vi "Proyecto Final.vi"() -> ()   [LabVIEW 2014]
panel:
  out "2061":string
  out "2060":string
  out "2059":string
  out "Datos Ambos":string
  out "Datos 2":string
  out "Datos 1":string
  in  "Modo":i16(slide) scale=1.0..5.0
  out "Motor 5":i64
  out "Motor 6":i64
  out "Motor 4":i64
  out "Motor 3":i64
  out "Motor 2":i64
  out "Motor 1":i64
  in  "reset":bool
  in  "?":bool
  in  "Motor 6":i64(knob) scale=-500.0..500.0
  in  "Motor 5":i64(knob) scale=-500.0..500.0
  in  "Motor 4":i64(knob) scale=-500.0..500.0
  in  "Motor 3":i64(knob) scale=-500.0..500.0
  in  "Motor 2":i64(knob) scale=-500.0..500.0
  in  "Motor 1":i64(knob) scale=-500.0..500.0
  # "Instrucciones:\nEn esta pantalla se pueden observar\n6 perillas, 6 indicadores y una barra \npara seleccionar el modo.\n\nBarra de Seleccion de Modo\nBrazo A LM: El leap motion enviara \nvalores del 0 al 5 para escoger una\nrutina predefinida en el brazo A\n\nBrazo B LM: El leap motion enviara \nvalores del 0 al 5 para escoger una\nrutina predefinida en el brazo B\n\nAmbos: Se controlaran ambos brazos\nal mismo tiempo\n\nBrazo A Manual: El brazo A tomará la\nposición que tengan las perillas\n\nBrazo B Manual: El brazo B tomará la\nposición que tengan las perillas"
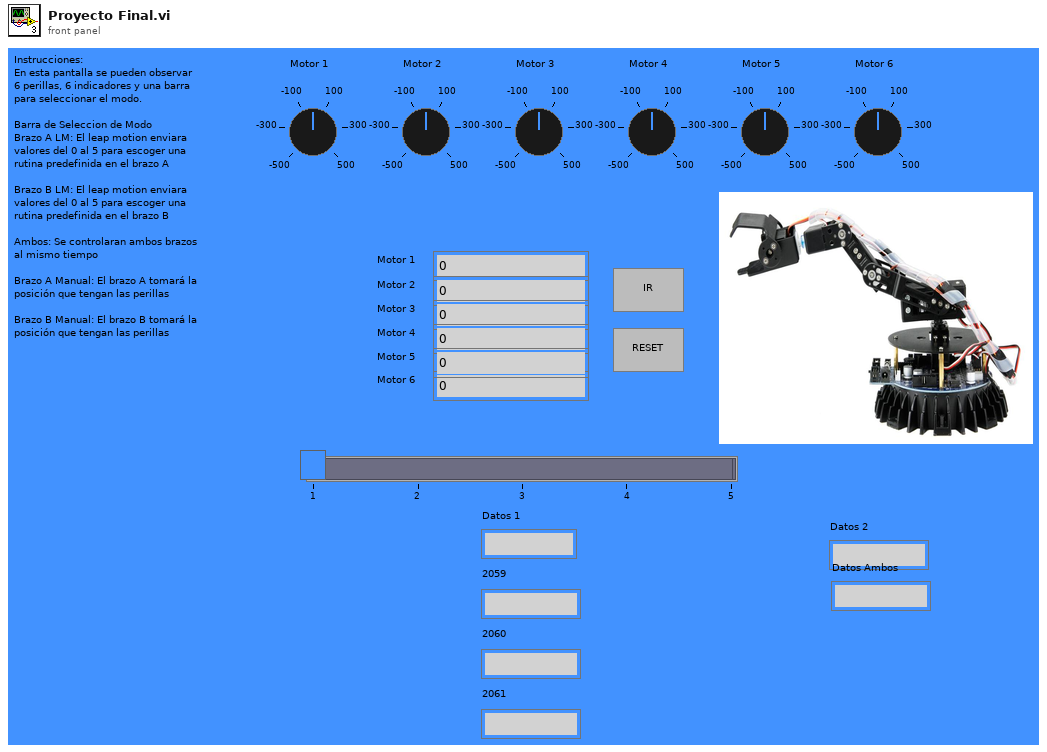
[diagram p1: front panel]
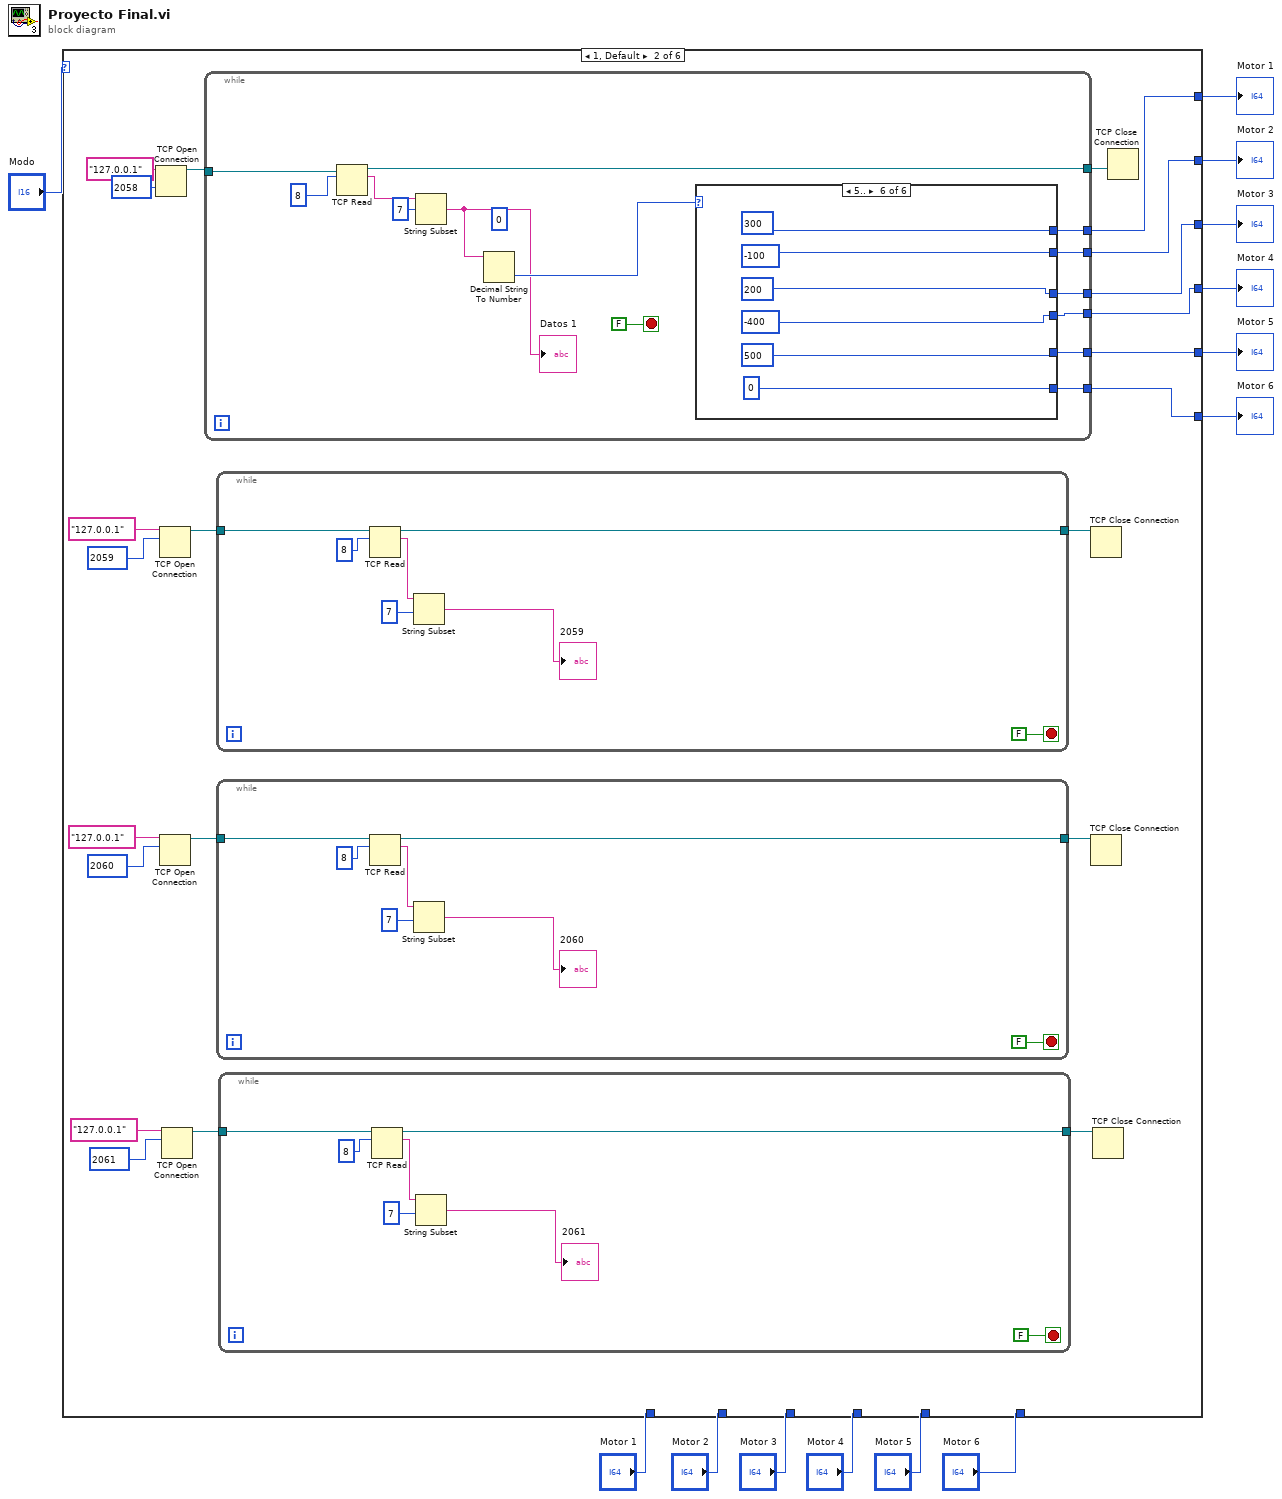
[diagram p0: block diagram]
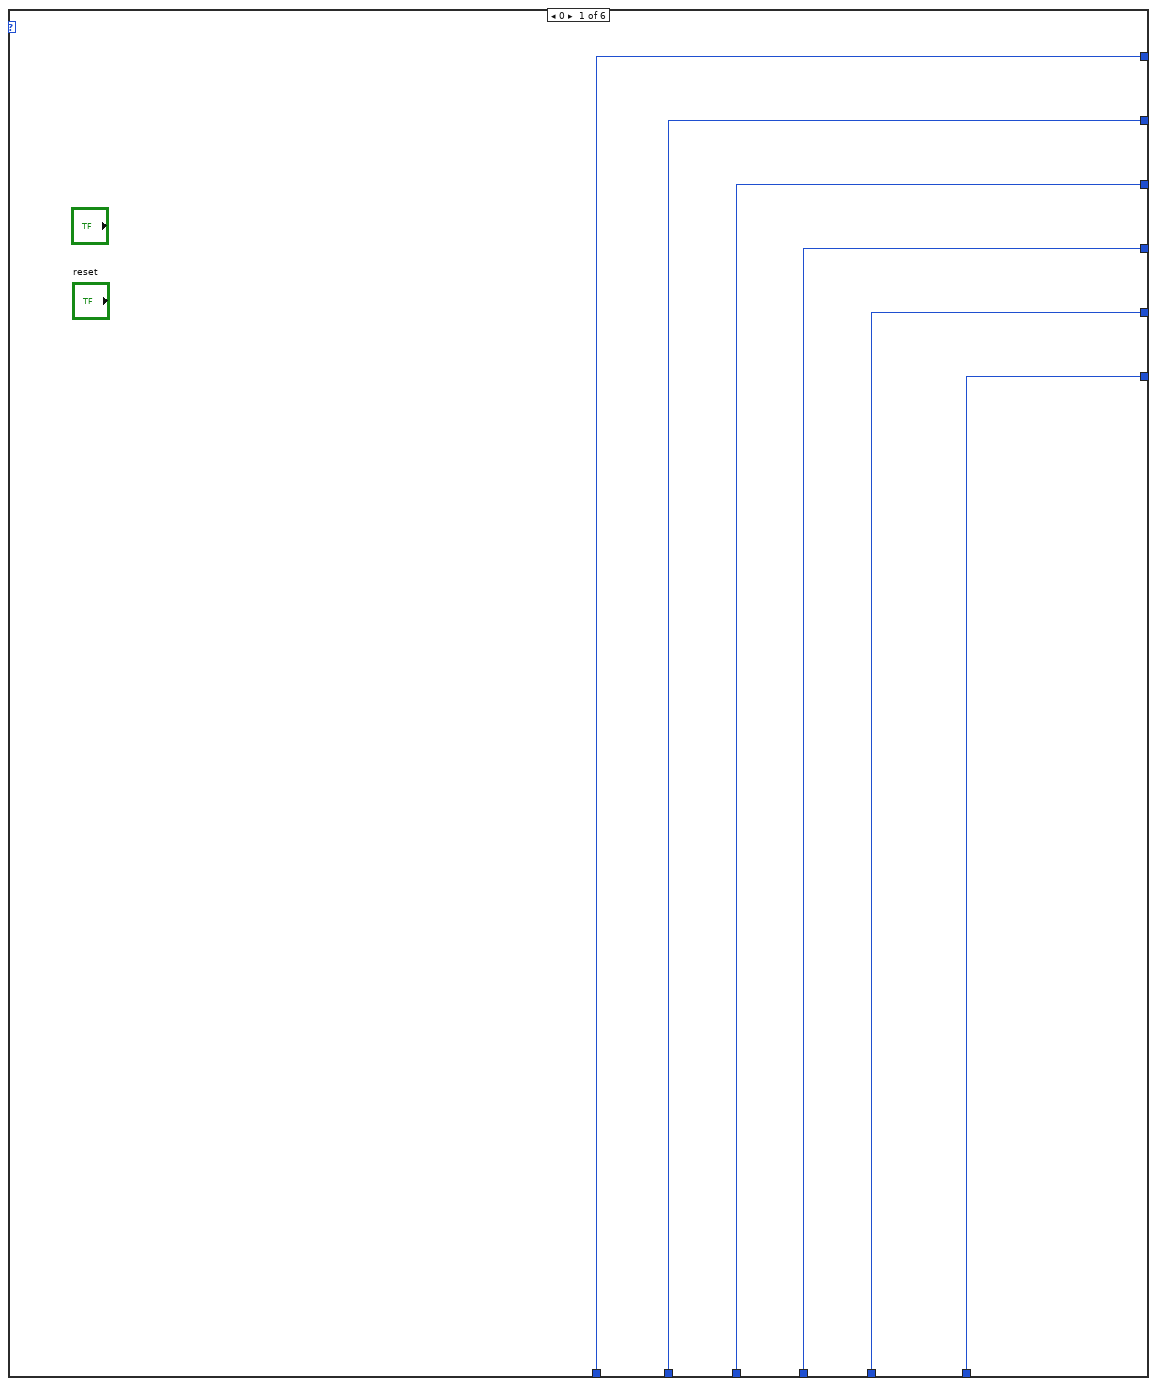
[diagram p2: hidden frame]
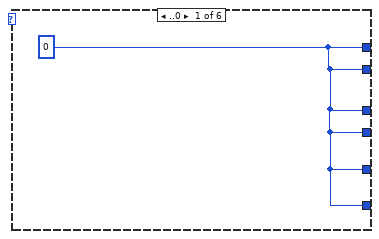
[diagram p3: hidden frame]
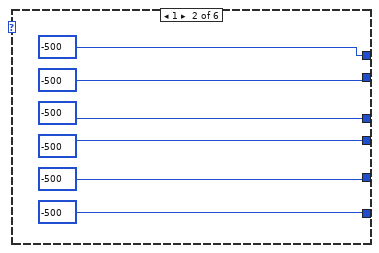
[diagram p4: hidden frame]
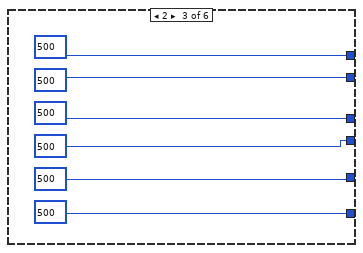
[diagram p5: hidden frame]
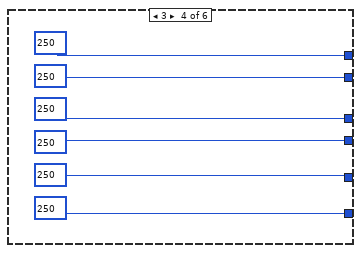
[diagram p6: hidden frame]
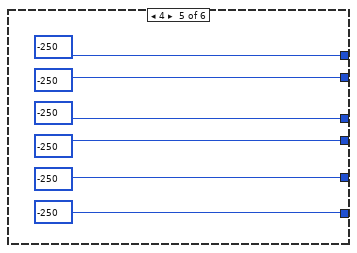
[diagram p7: hidden frame]
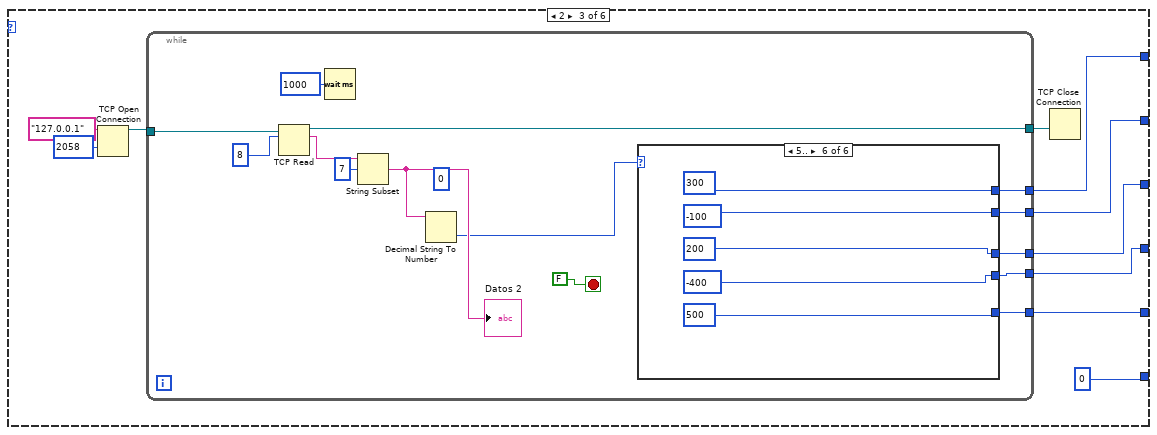
[diagram p8: hidden frame]
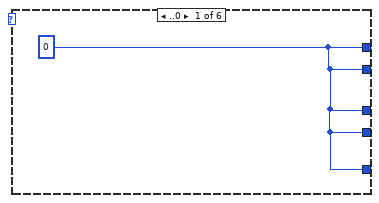
[diagram p9: hidden frame]
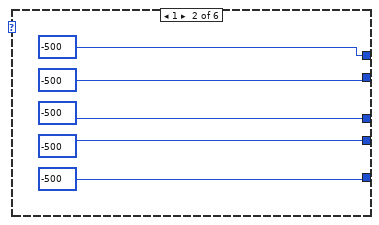
[diagram p10: hidden frame]
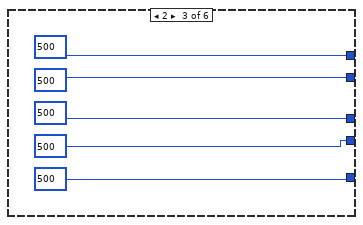
[diagram p11: hidden frame]
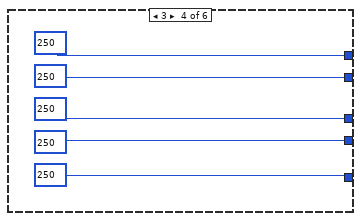
[diagram p12: hidden frame]
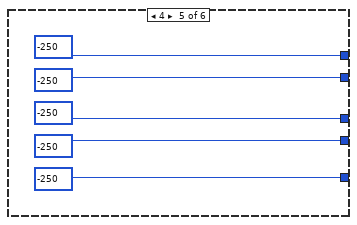
[diagram p13: hidden frame]
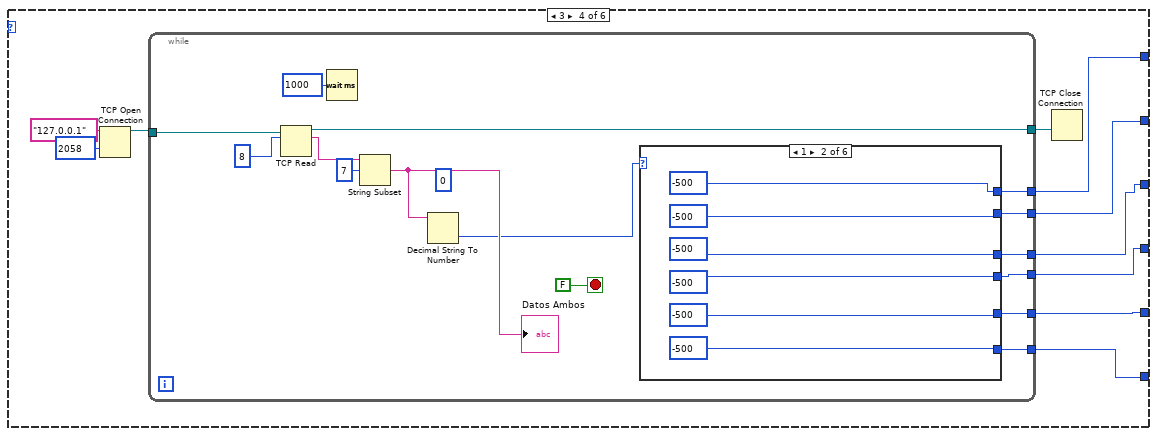
[diagram p14: hidden frame]
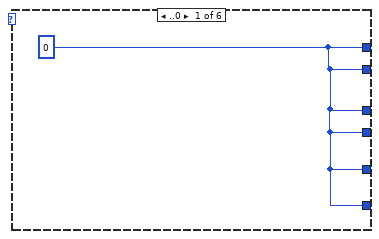
[diagram p15: hidden frame]
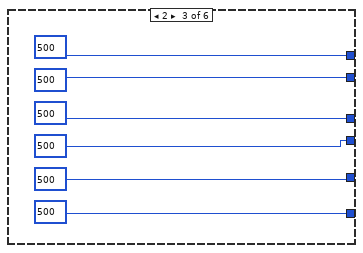
[diagram p16: hidden frame]
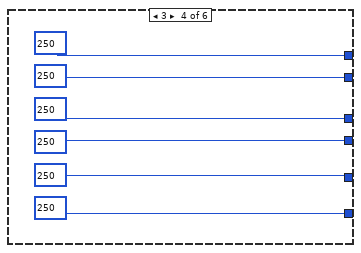
[diagram p17: hidden frame]
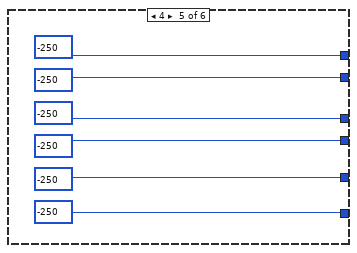
[diagram p18: hidden frame]
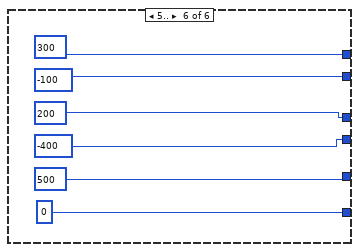
[diagram p19: hidden frame]
diagram:
  n1 = case shown="1, Default" "Modo" {
    tunnel: [w19 w37 w113 w163 w219 w225] -> w13
    tunnel: [w18 w36 w112 w162 w218 w224] -> w12
    tunnel: [w17 w35 w111 w161 w217 w223] -> w11
    tunnel: [w16 w34 w110 w160 w216 w222] -> w10
    tunnel: [w15 w33 w109 w159 w215 w221] -> w9
    tunnel: [w14 w32 0 w158 w214 0] -> w8
    tunnel: "Motor 1" -> [w19 _ _ _ w219 w225]
    tunnel: "Motor 2" -> [w18 _ _ _ w218 w224]
    tunnel: "Motor 3" -> [w17 _ _ _ w217 w223]
    tunnel: "Motor 4" -> [w16 _ _ _ w216 w222]
    tunnel: "Motor 5" -> [w15 _ _ _ w215 w221]
    tunnel: "Motor 6" -> [w14 _ _ _ w214 _]
    frame 0 {
    }
    frame 1, Default {
      n2 = TCP Open Connection(address="127.0.0.1", remote port or service name=u16 2058) -> (connection ID=w41:refnum<k5>)  [unwired: 3 in, 1 out]
      n3 = TCP Open Connection(address="127.0.0.1", remote port or service name=u16 2059) -> (connection ID=w29:refnum<k5>)  [unwired: 3 in, 1 out]
      n4 = TCP Open Connection(address="127.0.0.1", remote port or service name=u16 2060) -> (connection ID=w26:refnum<k5>)  [unwired: 3 in, 1 out]
      n5 = TCP Open Connection(address="127.0.0.1", remote port or service name=u16 2061) -> (connection ID=w21:refnum<k5>)  [unwired: 3 in, 1 out]
      n6 = while {
        tunnel: w41 -> [w76]
        tunnel: [w74] -> w38
        tunnel: [w71] -> w37
        tunnel: [w70] -> w36
        tunnel: [w69] -> w35
        tunnel: [w68] -> w34
        tunnel: [w67] -> w33
        tunnel: [w66] -> w32
        stop <- FALSE stop-if-true
        (unwired) 0 ("offset (0)")
        n7 = TCP Read(connection ID=w76, bytes to read=8) -> (connection ID out=w74:refnum<k5>, data out=w72:string)  [unwired: 3 in, 1 out]
        n8 = String Subset(string=w72, offset (0)=7) -> (substring=w64:string)  [unwired: 1 in]
        "Datos 1" <- w64
        n9 = Decimal String To Number(string=w64) -> (number=w65:i32)  [unwired: 2 in, 1 out]
        n10 = case shown="5.." w65 {
          tunnel: [w77 -500 500 250 -250 300] -> w71
          tunnel: [w77 -500 500 250 -250 -100] -> w70
          tunnel: [w77 -500 500 250 -250 200] -> w69
          tunnel: [w77 -500 500 250 -250 -400] -> w68
          tunnel: [w77 -500 500 250 -250 500] -> w67
          tunnel: [w77 -500 500 250 -250 0] -> w66
          frame ..0 {
            w77 = 0
          }
          frame 1 {
          }
          frame 2 {
          }
          frame 3 {
          }
          frame 4 {
          }
          frame 5.. {
          }
        }
      }
      n11 = while {
        tunnel: w29 -> [w62]
        tunnel: [w61] -> w28
        stop <- FALSE stop-if-true
        n12 = TCP Read(connection ID=w62, bytes to read=8) -> (connection ID out=w61:refnum<k5>, data out=w57:string)  [unwired: 3 in, 1 out]
        n13 = String Subset(string=w57, offset (0)=7) -> (substring=→"2059":string)  [unwired: 1 in]
      }
      n14 = while {
        tunnel: w26 -> [w55]
        tunnel: [w54] -> w27
        stop <- FALSE stop-if-true
        n15 = TCP Read(connection ID=w55, bytes to read=8) -> (connection ID out=w54:refnum<k5>, data out=w50:string)  [unwired: 3 in, 1 out]
        n16 = String Subset(string=w50, offset (0)=7) -> (substring=→"2060":string)  [unwired: 1 in]
      }
      n17 = while {
        tunnel: w21 -> [w48]
        tunnel: [w47] -> w20
        stop <- FALSE stop-if-true
        n18 = TCP Read(connection ID=w48, bytes to read=8) -> (connection ID out=w47:refnum<k5>, data out=w43:string)  [unwired: 3 in, 1 out]
        n19 = String Subset(string=w43, offset (0)=7) -> (substring=→"2061":string)  [unwired: 1 in]
      }
      n20 = TCP Close Connection(connection ID=w28) -> ()  [unwired: 2 in, 2 out]
      n21 = TCP Close Connection(connection ID=w27) -> ()  [unwired: 2 in, 2 out]
      n22 = TCP Close Connection(connection ID=w20) -> ()  [unwired: 2 in, 2 out]
      n23 = TCP Close Connection(connection ID=w38) -> ()  [unwired: 2 in, 2 out]
    }
    frame 2 {
      n24 = TCP Open Connection(address="127.0.0.1", remote port or service name=u16 2058) -> (connection ID=w117:refnum<k5>)  [unwired: 3 in, 1 out]
      n25 = while {
        tunnel: w117 -> [w131]
        tunnel: [w128] -> w114
        tunnel: [w125] -> w113
        tunnel: [w124] -> w112
        tunnel: [w123] -> w111
        tunnel: [w122] -> w110
        tunnel: [w121] -> w109
        stop <- FALSE stop-if-true
        (unwired) 0 ("offset (0)")
        n26 = TCP Read(connection ID=w131, bytes to read=8) -> (connection ID out=w128:refnum<k5>, data out=w126:string)  [unwired: 3 in, 1 out]
        n27 = Wait (ms)(milliseconds to wait=u32 1000) -> ()  [unwired: 1 out]
        n28 = String Subset(string=w126, offset (0)=7) -> (substring=w120:string)  [unwired: 1 in]
        "Datos 2" <- w120
        n29 = Decimal String To Number(string=w120) -> (number=w118:i32)  [unwired: 2 in, 1 out]
        n30 = case shown="5.." w118 {
          tunnel: [w132 -500 500 250 -250 300] -> w125
          tunnel: [w132 -500 500 250 -250 -100] -> w124
          tunnel: [w132 -500 500 250 -250 200] -> w123
          tunnel: [w132 -500 500 250 -250 -400] -> w122
          tunnel: [w132 -500 500 250 -250 500] -> w121
          frame ..0 {
            w132 = 0
          }
          frame 1 {
          }
          frame 2 {
          }
          frame 3 {
          }
          frame 4 {
          }
          frame 5.. {
          }
        }
      }
      n31 = TCP Close Connection(connection ID=w114) -> ()  [unwired: 2 in, 2 out]
    }
    frame 3 {
      n32 = TCP Open Connection(address="127.0.0.1", remote port or service name=u16 2058) -> (connection ID=w167:refnum<k5>)  [unwired: 3 in, 1 out]
      n33 = while {
        tunnel: w167 -> [w182]
        tunnel: [w179] -> w164
        tunnel: [w176] -> w163
        tunnel: [w175] -> w162
        tunnel: [w174] -> w161
        tunnel: [w173] -> w160
        tunnel: [w172] -> w159
        tunnel: [w171] -> w158
        stop <- FALSE stop-if-true
        (unwired) 0 ("offset (0)")
        n34 = TCP Read(connection ID=w182, bytes to read=8) -> (connection ID out=w179:refnum<k5>, data out=w177:string)  [unwired: 3 in, 1 out]
        n35 = Wait (ms)(milliseconds to wait=u32 1000) -> ()  [unwired: 1 out]
        n36 = String Subset(string=w177, offset (0)=7) -> (substring=w170:string)  [unwired: 1 in]
        "Datos Ambos" <- w170
        n37 = Decimal String To Number(string=w170) -> (number=w168:i32)  [unwired: 2 in, 1 out]
        n38 = case shown="1" w168 {
          tunnel: [w183 -500 500 250 -250 300] -> w176
          tunnel: [w183 -500 500 250 -250 -100] -> w175
          tunnel: [w183 -500 500 250 -250 200] -> w174
          tunnel: [w183 -500 500 250 -250 -400] -> w173
          tunnel: [w183 -500 500 250 -250 500] -> w172
          tunnel: [w183 -500 500 250 -250 0] -> w171
          frame ..0 {
            w183 = 0
          }
          frame 1 {
          }
          frame 2 {
          }
          frame 3 {
          }
          frame 4 {
          }
          frame 5.. {
          }
        }
      }
      n39 = TCP Close Connection(connection ID=w164) -> ()  [unwired: 2 in, 2 out]
    }
    frame 4 {
    }
    frame 5 {
    }
  }
  "Motor 2" <- w12
  "Motor 3" <- w11
  "Motor 4" <- w10
  "Motor 6" <- w8
  "Motor 5" <- w9
  "Motor 1" <- w13
